vi "DMD 2 Display.vi"() -> ()   [LabVIEW 2020]
uses:
  <vilib>/Utility/miscctls.llb/LVPointTypeDef.ctl
  <vilib>/Utility/miscctls.llb/LVBoundsTypeDef.ctl
  <vilib>/Utility/miscctls.llb/LVRectTypeDef.ctl
panel:
  in  "Monitor":u16
  in  "8-bit pixmap":u8[][](array[numeric])
  out "PictureBox":picture
  in  "stop":bool
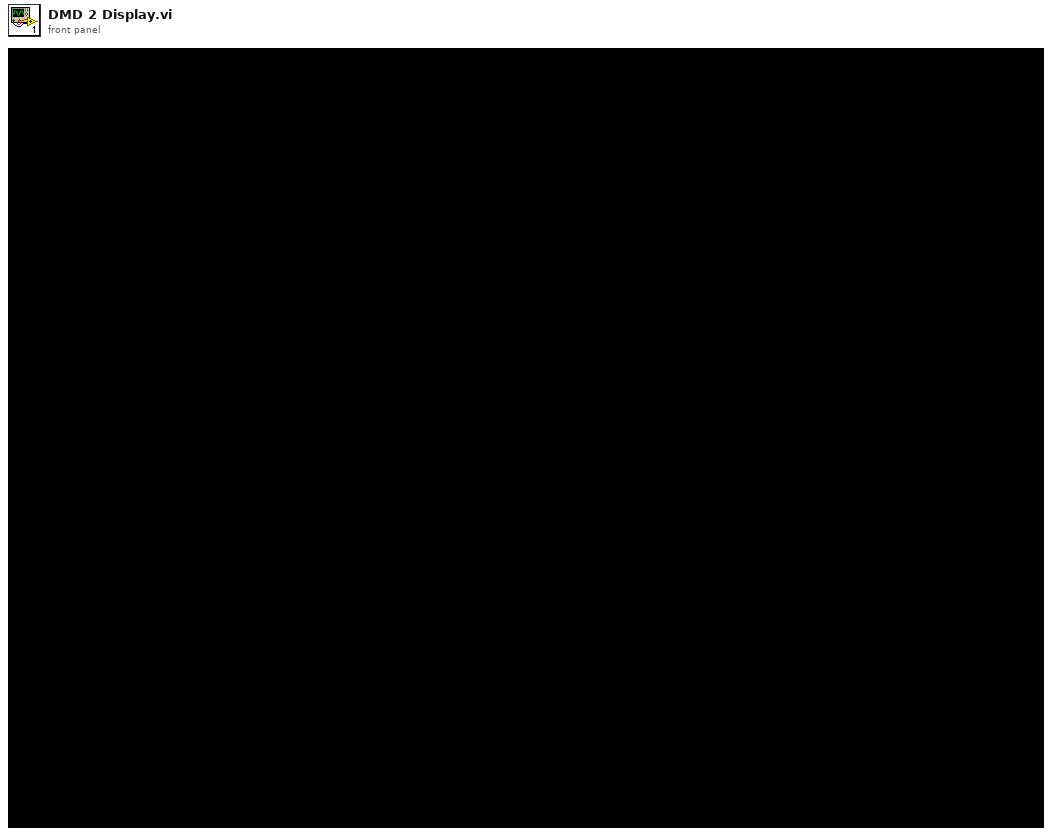
[diagram p1: front panel]
types:
  T1 = typedef "LVRectTypeDef.ctl" = cluster{"Left":i16, "Top":i16, "Right":i16, "Bottom":i16}
  T2 = typedef "LVBoundsTypeDef.ctl" = cluster{"Width":u32, "Height":u32}
  T3 = typedef "LVPointTypeDef.ctl" = cluster{"Horizontal":i16, "Vertical":i16}
  T4 = typedef "imagedata.ctl" = cluster{"image type":i32, "image depth":i32, "image":u8[], "mask":u8[], "colors":u32[], "Rectangle":cluster{"left":i16, "top":i16, "right":i16, "bottom":i16}}
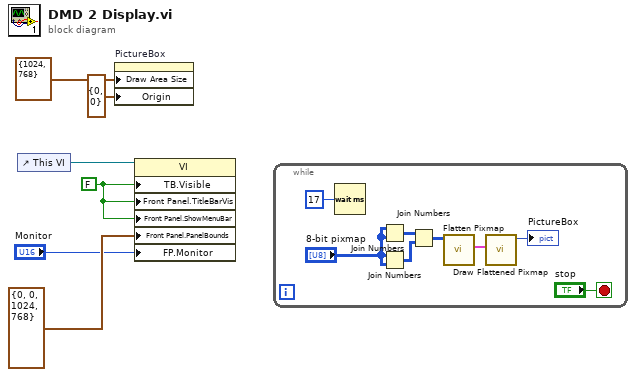
[diagram p0: block diagram]
diagram:
  w3 = FALSE ("Tool Bar:Visible")
  n1 = control-ref of="This VI"() -> (w4:refnum<vi>)
  n2 = property on="PictureBox" class="Pict"("Draw Area Size"=T2 {"Width"=1024, "Height"=768}, "Origin"=T3 {"Horizontal"=0, "Vertical"=0}) -> ()  [unwired: 2 in, 2 out]
  n3 = property class="VI"(reference=w4, "TB.Visible"=w3, "Front Panel.TitleBarVis"=w3, "Front Panel.ShowMenuBar"=w3, "Front Panel.PanelBounds"=T1 {"Left"=0, "Top"=0, "Right"=1024, "Bottom"=768} ("Front Panel Window:Panel Bounds"), "FP.Monitor"="Monitor") -> ()  [unwired: 1 in, 2 out]
  n4 = while {
    stop <- "stop" stop-if-true
    n5 = Wait (ms)(milliseconds to wait=u32 17) -> ()  [unwired: 1 out]
    n6 = Join Numbers(hi="8-bit pixmap", lo="8-bit pixmap") -> ((hi.lo)=w9:u16[][])
    n7 = Join Numbers(hi="8-bit pixmap", lo="8-bit pixmap") -> ((hi.lo)=w8:u16[][])
    n8 = Join Numbers(hi=w9, lo=w8) -> ((hi.lo)=w7:u32[][])
    n9 = call <vilib>:"Flatten Pixmap.vi"("24-bit pixmap"=w7) -> ("image data"=w13:T4)  [unwired: 10 in]
    n10 = call <vilib>:"Draw Flattened Pixmap.vi"("image data"=w13) -> ("new picture"=→"PictureBox":picture)  [unwired: 8 in]
  }
